vi "Write Points.vi"(8 "error in (no error)":errorcluster, 10 "Points":cluster{"X":dbl, "Y":dbl}[](array[cluster]), 11 "Tool Object in":refnum<class "Tool Object.lvclass">) -> (0 "error out":errorcluster, 3 "Tool Object out":refnum<class "Tool Object.lvclass">)   [LabVIEW 2019, in "Tool Object.lvclass"]
uses:
  Tool Object.lvclass
  Tool Object.lvclass/Tool Object.ctl
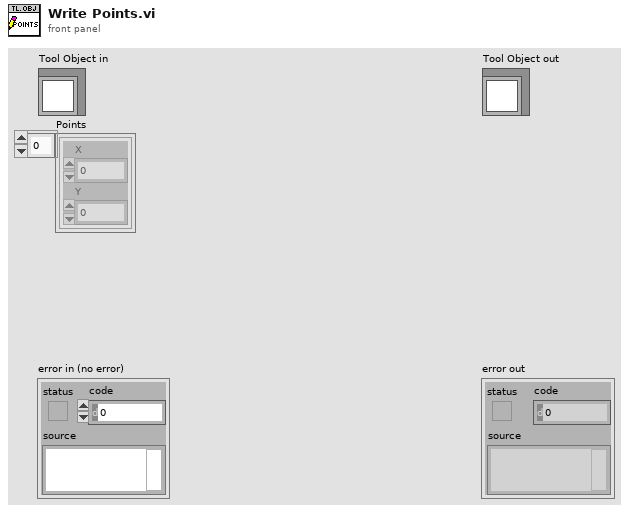
[diagram p1: front panel]
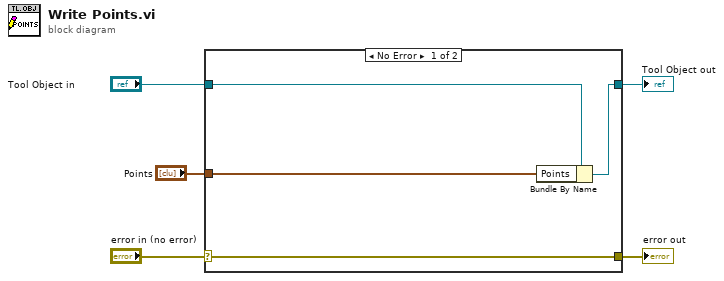
[diagram p0: block diagram]
diagram:
  n1 = case shown="No Error" "error in (no error)" {
    selector: "error in (no error)" -> [w9 w10]
    tunnel: [w9 w10] -> w4
    tunnel: [w7 w11] -> w2
    tunnel: "Tool Object in" -> [w8 w11]
    tunnel: "Points" -> [w6 _]
    frame No Error {
      n2 = Bundle By Name(cluster=w8, "Points"=w6) -> (w7:refnum<class "Tool Object.lvclass">)
    }
    frame Error {
    }
  }
  "error out" <- w4
  "Tool Object out" <- w2
